vi "Get Available Base System Images.vi"(8 "error in (no error)":errorcluster, 11 "Session in":refnum<k21>) -> (0 "error out":errorcluster, 2 "Base System Images":T1[](array[typedef]) {"component type" items=["standard", "hidden", "system", "unknown", "startup", "image", "essential"]}, 3 "Session out":refnum<k21>)   [LabVIEW 2020, in "nisyscfg.lvlib"]
doc: "Retrieves a collection of base system images that are available for installation to the specified target."
uses:
  <vilib>/nisyscfg/nisyscfg.lvlib
  <vilib>/nisyscfg/Software 1.2.ctl
  <vilib>/nisyscfg/Component Type.ctl
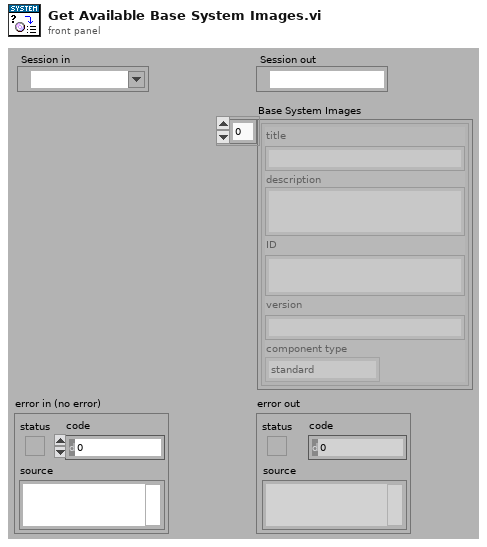
[diagram p1: front panel]
types:
  T1 = typedef "nisyscfg.lvlib/Software 1.2.ctl" = cluster{"title":string, "description":string, "ID":string, "version":string, "component type":T2}
  T2 = typedef "nisyscfg.lvlib/Component Type.ctl" = u32
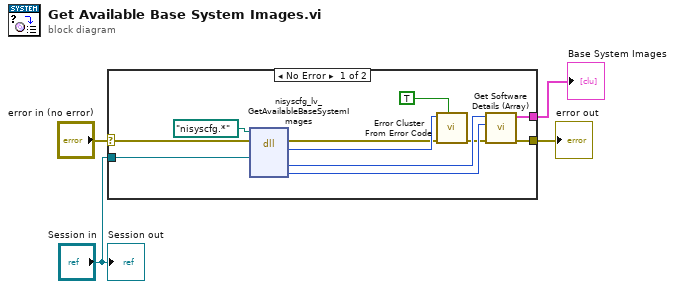
[diagram p0: block diagram]
diagram:
  n1 = case shown="No Error" "error in (no error)" {
    selector: "error in (no error)" -> [w13 w16]
    tunnel: [w6 w16] -> w4
    tunnel: "Session in" -> [w12 _]
    tunnel: [w5 _] -> w1
    frame No Error {
      n2 = dll-call lib="nisyscfg.*" fn="nisyscfg_lv_GetAvailableBaseSystemImages" label="GetAvailableBaseSystemImages"(path in=path "nisyscfg.*", error in=w13, "system"=w12) -> (error out=w14:errorcluster, "result"=w15:i32, "systemImages"=w9:u64, "numSystemImages"=w8:i32)  [unwired: 4 in, 1 out]
      n3 = call <vilib>:"Error Cluster From Error Code.vi"("show call chain? (False)"=TRUE, "error in (no error)"=w14, "error code (0)"=w15) -> ("error out"=w7:errorcluster)  [unwired: 6 in]
      n4 = call <vilib>:"Get Software Details (Array).vi"("error in (no error)"=w7, "Number of Elements"=w8, "Enumerator in"=w9) -> ("error out"=w6:errorcluster, "Software Components"=w5:T1[])  [unwired: 7 in]
    }
    frame Error {
    }
  }
  "error out" <- w4
  "Base System Images" <- w1
  "Session out" <- "Session in"
